vi "PhotonCamera_VerifyVersion.vi"(11 "BaseNTName":string="/photonvision") -> (0 "error out":errorcluster, 3 "VersionOk":bool)   [LabVIEW 2019, in "PhotonVisionLib.lvlib"]
doc: "Verify photonvision version string\n\nCurrently this does not write a driver station message if the version is wrong.\n\nInputs:\n - BaseNTName - string - Base Nework Table name. (Optional. Default: /photonvision )\n \nOutputs:\n - VersionOk - string - Version matches co-processor.\n - Error Out -- Contains error information if a Network table ot other error occured."
uses:
  PhotonVisionLib.lvlib
  <vilib>/Rock Robotics/Network Tables/NT Read String.vi
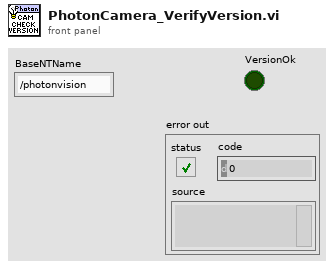
[diagram p1: front panel]
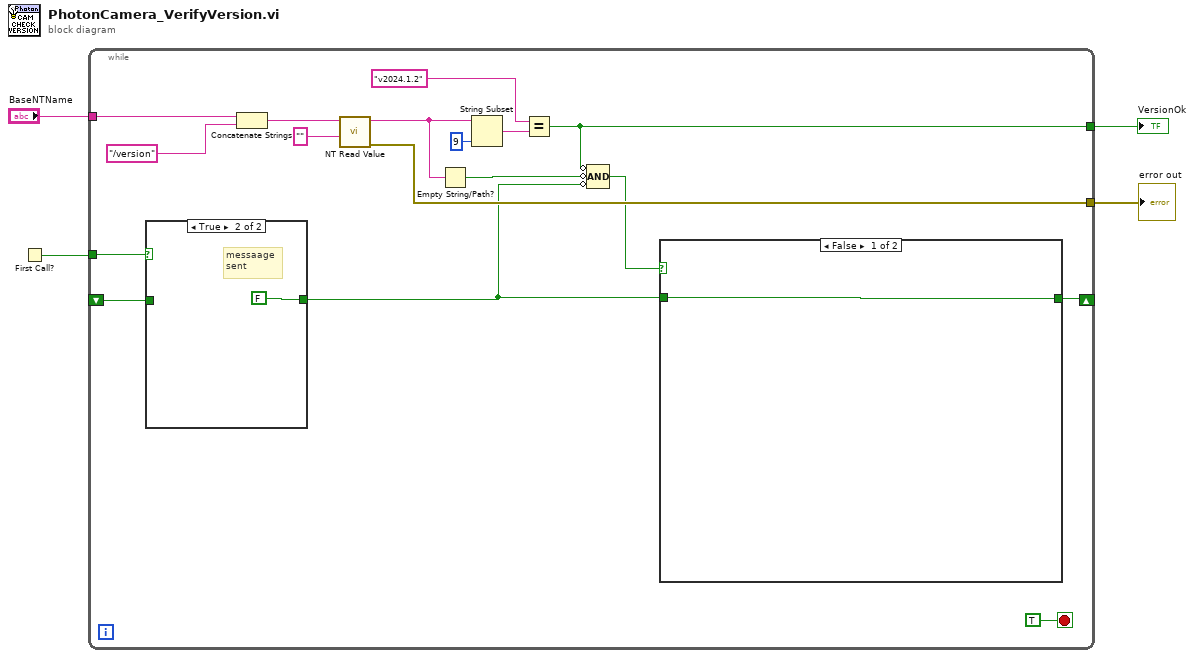
[diagram p0: block diagram]
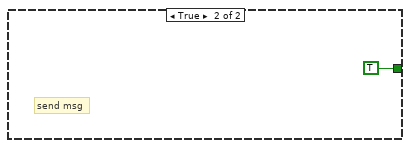
[diagram p2: hidden frame]
diagram:
  n1 = First Call?() -> (First Call?: T/F=w1:bool)
  n2 = while {
    tunnel: [w21] -> w4
    tunnel: "BaseNTName" -> [w18]
    tunnel: w1 -> [w12]
    shift-right: [w5] -> _
    shift-left: _ -> [w11]
    tunnel: [w9] -> w2
    stop <- TRUE stop-if-true
    n3 = case shown="True" w12 {
      tunnel: [w24 FALSE] -> w6
      tunnel: w11 -> [w24 _]
      frame False {
      }
      frame True {
        # "messaage \nsent"
      }
    }
    n4 = Concatenate Strings(w18, "/version") -> (w17:string)
    n5 = call-poly <vilib>:"NT Read Value.vi"("default value"="", "name"=w17) -> ("error out"=w21:errorcluster, "value"=w10:string)  [unwired: 7 in, 1 out]
    n6 = Empty String/Path?(string/path=w10) -> (empty?=w8:bool)
    n7 = String Subset(string=w10, length (rest)=9 ("length (rest)")) -> (substring=w14:string)  [unwired: 1 in]
    n8 = Equal?(x="v2024.1.2", y=w14) -> (x = y?=w9:bool)
    n9 = Compound Arithmetic op=AND(invert w9, invert w8, invert w6) -> (w7:bool)
    n10 = case shown="False" w7 {
      tunnel: w6 -> [w22 _]
      tunnel: [w22 TRUE] -> w5
      frame False {
      }
      frame True {
        # "send msg"
      }
    }
  }
  "error out" <- w4
  "VersionOk" <- w2
